vi "Recursive find VIs.vi"(8 "error in (no error)":errorcluster, 11 "Project Items":refnum<vi>[](array[refnum])) -> (0 "error out":errorcluster, 3 "VIs":set{path}(c389))   [LabVIEW 2020, in "Coverage Analyzer.lvclass"]
uses:
  Coverage Analyzer.lvclass
  a1401d1e-ec1c-4a27-9029-e4c0d22f2509.vi
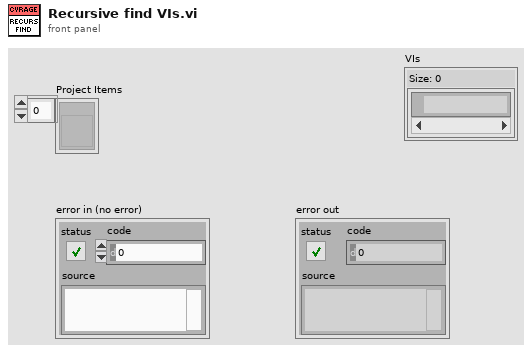
[diagram p1: front panel]
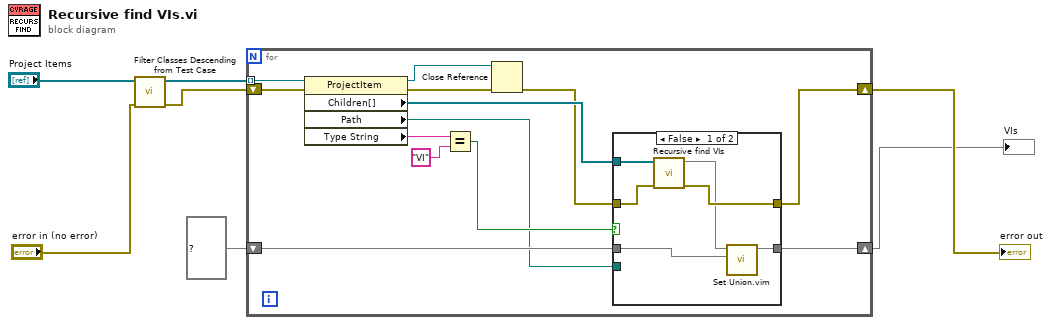
[diagram p0: block diagram]
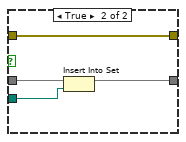
[diagram p2: hidden frame]
diagram:
  n1 = call "Filter Classes Descending from Test Case.vi"("error in (no error)"="error in (no error)", "Project Items"="Project Items") -> ("error out"=w1:errorcluster, "Project Items out"=w3:refnum<vi>[])  [unwired: 8 in]
  n2 = for {
    tunnel: w3 -> [w17] mode=indexing
    shift-right: [w11] -> w7
    shift-left: w1 -> [w16]
    shift-right: [w9] -> w5
    shift-left: set{path} {} ("VIs") -> [w10]
    n3 = property class="ProjectItem"(reference=w17, error in=w16) -> (reference out=w14:refnum<vi>, error out=w15:errorcluster, "Children[]"=w13:refnum<vi>[], "Path"=w8:path, "Type String"=w20:string)
    n4 = Equal?(x=w20, y="VI") -> (x = y?=w18:bool)
    n5 = Close Reference(reference=w14, error in (no error)=w15) -> (error out=w12:errorcluster)
    n6 = case shown="False" w18 {
      tunnel: w13 -> [w26 _]
      tunnel: [w21 w29] -> w9
      tunnel: w12 -> [w25 w30]
      tunnel: [w24 w30] -> w11
      tunnel: w10 -> [w22 w28]
      tunnel: w8 -> [_ w27]
      frame False {
        n7 = call "Recursive find VIs.vi"("error in (no error)"=w25, "Project Items"=w26) -> ("error out"=w24:errorcluster, "VIs"=w23:set{path})  [unwired: 8 in]
        n8 = call "Set Union.vim"("set 2"=w22, "set 1"=w23) -> ("union"=w21:set{path})  [unwired: 9 in]
      }
      frame True {
        n9 = Insert Into Set(10:w27, 11:w28) -> (3:w29:set{path})  [unwired: 1 out]
      }
    }
  }
  "error out" <- w7
  "VIs" <- w5
